vi "evaluate_SP.vi"(4 "lo_limit":dbl, 5 "hi_limit":dbl=50.0, 6 "lo_warn":dbl=5.0, 7 "hi_warn":dbl=45.0, 10 "F_O_now":dbl=30.0, 11 "change":dbl) -> (0 "status":u32(colorbox), 2 "F_O_new":dbl)   [LabVIEW 2019]
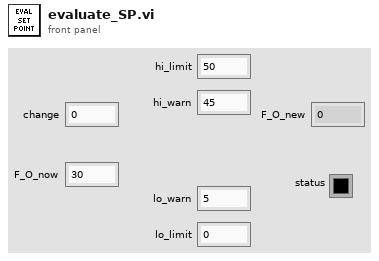
[diagram p1: front panel]
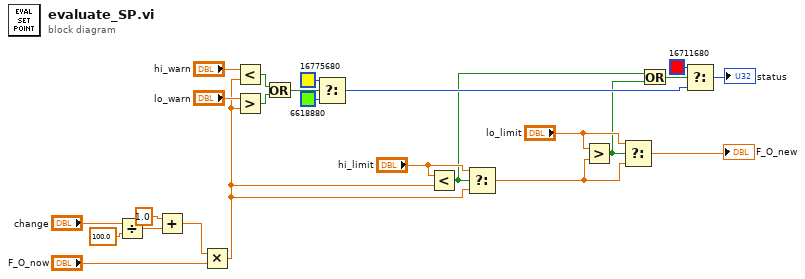
[diagram p0: block diagram]
diagram:
  n1 = Divide(x="change", y=100.0) -> (x/y=w21:dbl)
  n2 = Add(x=1.0, y=w21) -> (x+y=w19:dbl)
  n3 = Multiply(x=w19, y="F_O_now") -> (x*y=w11:dbl)
  n4 = Less?(x="hi_warn", y=w11) -> (x < y?=w9:bool)
  n5 = Greater?(x="lo_warn", y=w11) -> (0:w10:bool)
  n6 = Or(x=w9, y=w10) -> (x .or. y?=w8:bool)
  n7 = Select(t=u32 16775680 ("alarm_status"), s=w8, f=u32 6618880 ("alarm_status")) -> (s? t:f=w13:u32)
  n8 = Less?(x="hi_limit", y=w11) -> (x < y?=w4:bool)
  n9 = Select(t="hi_limit", s=w4, f=w11) -> (s? t:f=w6:dbl)
  n10 = Greater?(x="lo_limit", y=w6) -> (0:w3:bool)
  n11 = Select(t="lo_limit", s=w3, f=w6) -> (s? t:f=→"F_O_new":dbl)
  n12 = Or(x=w4, y=w3) -> (x .or. y?=w2:bool)
  n13 = Select(t=u32 16711680 ("alarm_status"), s=w2, f=w13) -> (s? t:f=→"status":u32)
